vi "String to Data Type.vi"(8 "error in (no error)":errorcluster, 11 "String":string) -> (0 "error out":errorcluster, 3 "Boolean out":refnum<class "String.lvclass">)   [LabVIEW 2020, in "String.lvclass"]
uses:
  <vilib>/gpm_packages/@cs/data-type-serializer/source/String/String.lvclass
  <vilib>/gpm_packages/@cs/data-type-serializer/source/String/String.lvclass/String.ctl
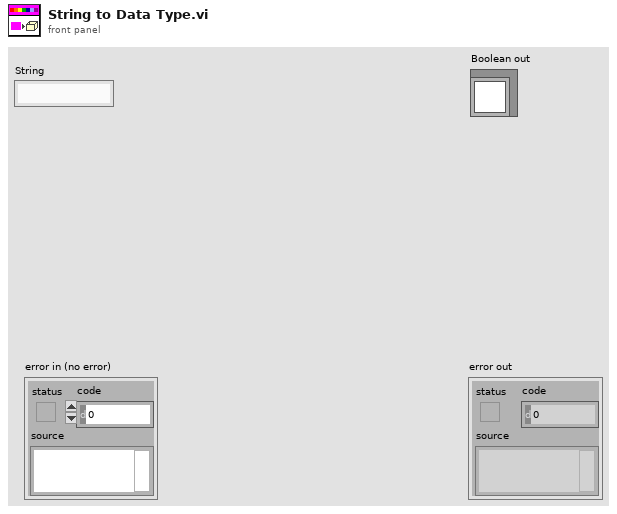
[diagram p1: front panel]
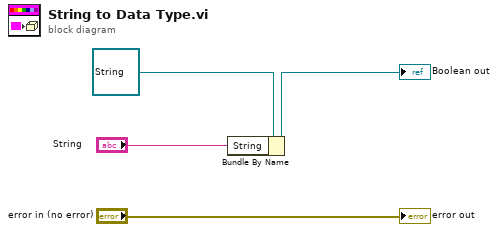
[diagram p0: block diagram]
diagram:
  n1 = Bundle By Name(cluster=refnum<class "String.lvclass"> refnum ("Boolean in"), "String"="String") -> (→"Boolean out":refnum<class "String.lvclass">)
  "error out" <- "error in (no error)"
